vi "Initialize From Settings.vi"(8 "error in (no error)":errorcluster, 9 "settings version":T1, 10 "settings":cluster{"key":string, "value":string}[](array[cluster]), 11 "Core Plugins Configuration in":refnum<class "Core Plugin Configuration.lvclass">) -> (0 "error out":errorcluster, 3 "Core Plugins Configuration out":refnum<class "Core Plugin Configuration.lvclass">)   [LabVIEW 2017, in "DSF Core.lvlib" / "Core Plugin Configuration.lvclass"]
uses:
  Core Plugin Configuration.lvclass
  Typedefs/DSF Version Info.ctl
  Core Plugin Configuration.lvclass/Core Plugin Configuration.ctl
  DSF Core.lvlib
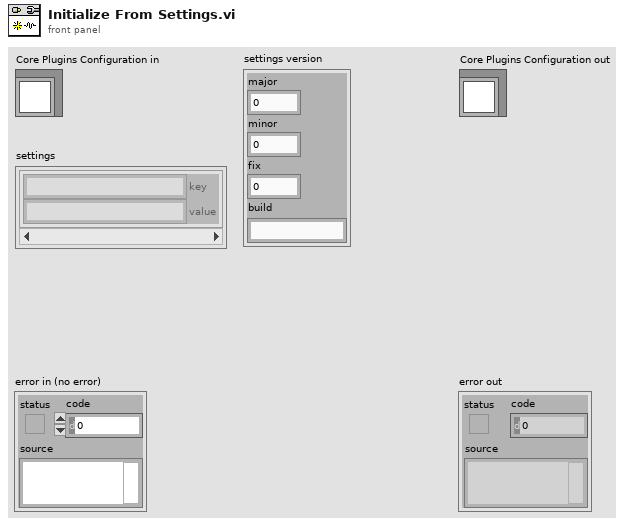
[diagram p1: front panel]
types:
  T1 = typedef "DSF Core.lvlib/DSF Version Info.ctl" = cluster{"major":u32, "minor":u32, "fix":u32, "build":string}
  T2 = cluster{"name":string, "components":string[], "cycle timing":cluster{"priority":u64, "decimation":u64, "offset":u64}}
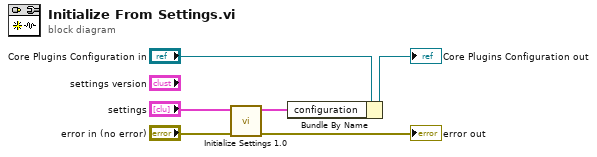
[diagram p0: block diagram]
diagram:
  n1 = call "Initialize Settings 1.0.vi"("error in (no error)"="error in (no error)", "settings 1.0"="settings") -> ("error out"=→"error out":errorcluster, "configuration 1.0"=w2:T2)  [unwired: 8 in]
  n2 = Bundle By Name(cluster="Core Plugins Configuration in", "configuration"=w2) -> (→"Core Plugins Configuration out":refnum<class "Core Plugin Configuration.lvclass">)
